vi "GUI_HTU_EMQ_triplet v2.vi"() -> ()   [LabVIEW 2020]
uses:
  Shared/GUI_Template/GUI_master/tcp_new_data_event.ctl
  Shared/GUI_Template/GUI_master/tcp new data cluster.ctl
panel:
  in  "Polarity_Switch.Ch3::1":enum16{"on", "off"}(ring) caption="Enable EMQ3"
  in  "Polarity_Switch.Ch2::1":enum16{"on", "off"}(ring) caption="Enable EMQ2"
  in  "Polarity_Switch.Ch1::1":enum16{"on", "off"}(ring) caption="Enable EMQ1"
  out "Chart":cluster{dbl, dbl, dbl}(graph)
  out "EMQ3 indicator":bool
  out "EMQ2 indicator":bool
  out "EMQ1 indicator":bool
  in  "SwitchWait":dbl=1500.0 min=0.0 max=12.0
  in  "CurrentSwitch limit":dbl=0.03 min=0.0 max=12.0
  out "Power.Ch2::1":dbl caption="Power::2" min=0.0 max=12.0
  out "Voltage.Ch2::1":dbl caption="Voltage::2" min=0.0 max=12.0
  out "Current.Ch2::1":dbl caption="Current::2" min=0.0 max=12.0
  out "Power.Ch3::1":dbl caption="Power::3" min=0.0 max=12.0
  out "Voltage.Ch3::1":dbl caption="Voltage::3" min=0.0 max=12.0
  out "Current.Ch3::1":dbl caption="Current::3" min=0.0 max=12.0
  out "Power.Ch1::1":dbl caption="Power::1" min=0.0 max=12.0
  out "Voltage.Ch1::1":dbl caption="Voltage::1" min=0.0 max=12.0
  out "Current.Ch1::1":dbl caption="Current::1" min=0.0 max=12.0
  in  "Voltage_Limit.Ch3::1":dbl caption="EMQ3 Voltage" min=0.0 max=12.0
  in  "Enable_Output.Ch3::1":enum16{"on", "off"}(ring) caption="Enable EMQ3"
  in  "Current_Limit.Ch3::1":dbl caption="EMQ3 Current" min=-10.0 max=10.0
  in  "Voltage_Limit.Ch1::1":dbl caption="EMQ1 Voltage" min=0.0 max=12.0
  in  "Voltage_Limit.Ch2::1":dbl caption="EMQ2 Voltage" min=0.0 max=12.0
  in  "Enable_Output.Ch2::1":enum16{"on", "off"}(ring) caption="Enable EMQ2"
  in  "Enable_Output.Ch1::1":enum16{"on", "off"}(ring) caption="Enable EMQ1"
  in  "Current_Limit.Ch1::1":dbl caption="EMQ1 Current" min=-10.0 max=10.0
  in  "Current_Limit.Ch2::1":dbl caption="EMQ2 Current" min=-10.0 max=10.0
  in  "UDP error message":string
  in  "GUIdevice 1":string="U_EMQTripletBipolar"
  out "error IO 2":errorcluster
  out "tcp data event":T1
  in  "stop":bool
  # "HTU EMQ Triplet"
  # "Polarity indicator"
  # "EMQ1\nEMQ1"
  # "EMQ2\nEMQ2"
  # "EMQ3"
  # "Enable output"
  # "Current Limit"
  # "Voltage Limit"
  # "Current"
  # "Voltage"
  # "Power"
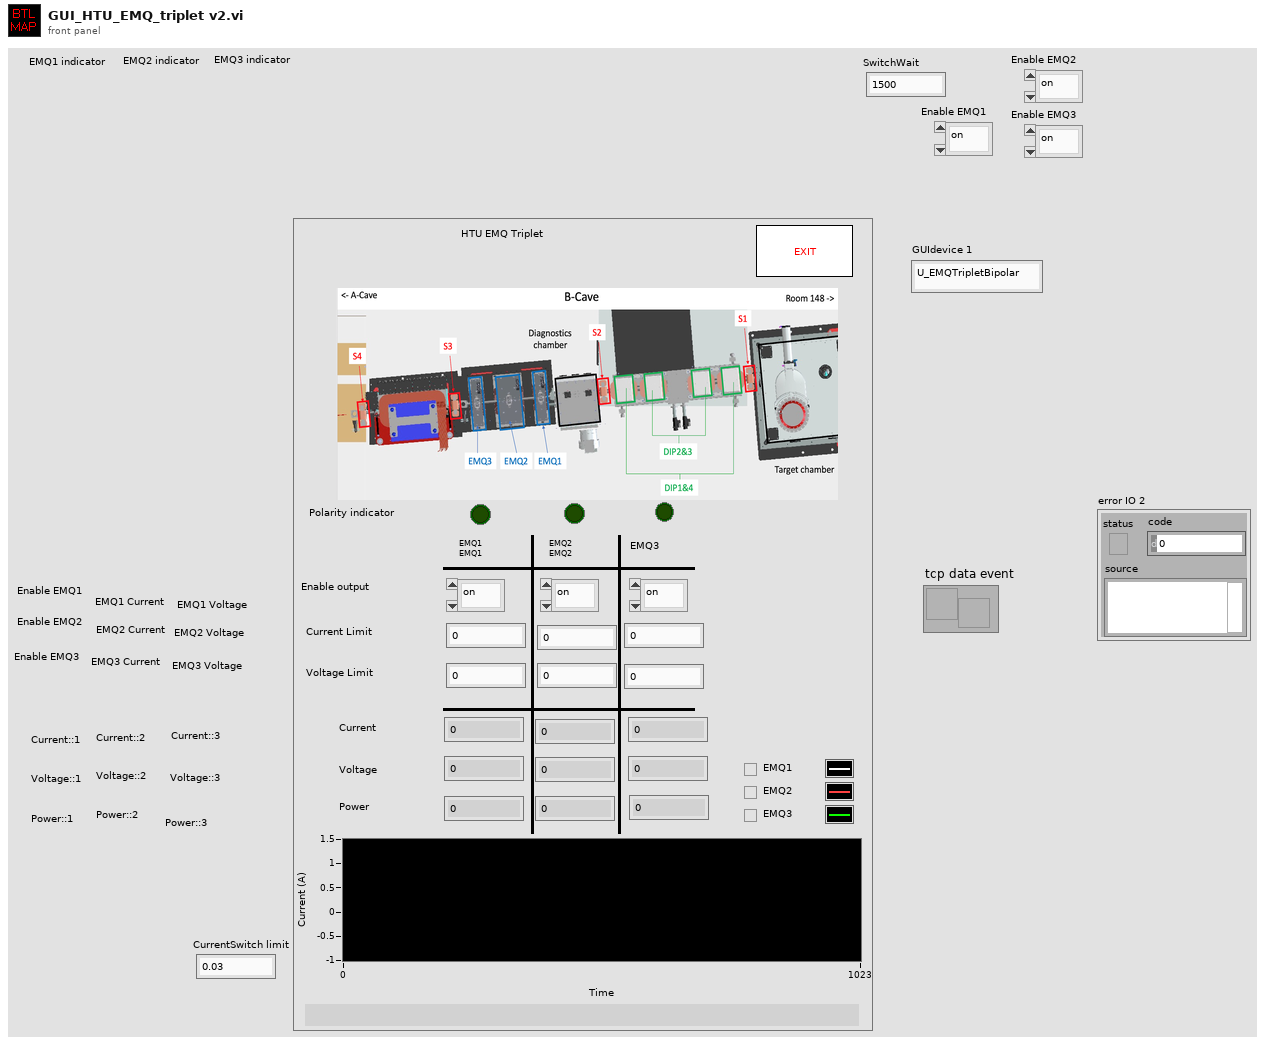
[diagram p1: front panel]
types:
  T1 = typedef "tcp_new_data_event.ctl" = refnum<user-event>
  T2 = typedef "tcp new data cluster.ctl" = cluster{"EventEnum":enum16{"new data", "connection status update"}, "Device name":string}
  T3 = enum32{"invalid app kind", "Development System", "Run Time System", "Student Edition", "Embedded LabVIEW", "Evaluation", "Custom"}
  T4 = enum32{"Invalid", "Standard", "Closed", "Hidden", "Minimized", "Maximized"}
  T5 = cluster{"Core":cluster{"Current VI Reference":refnum<vi>, "Close Panel on Exit?":bool}, "CurrentGraph1":dbl[][], "EMQ1PolaritySwitched":bool, "EMQ2PolaritySwitched":bool, "EMQ3PolaritySwitched":bool, "DegaussEMQ1":bool, "degauss loop":i32, "EMQ1DegaussSetCur":dbl, "EMQ2DegaussSetCur":dbl, "EMQ3DegaussSetCur":dbl, "last chart update tck":i32}
  T6 = cluster{"Current VI Reference":refnum<vi>, "Close Panel on Exit?":bool}
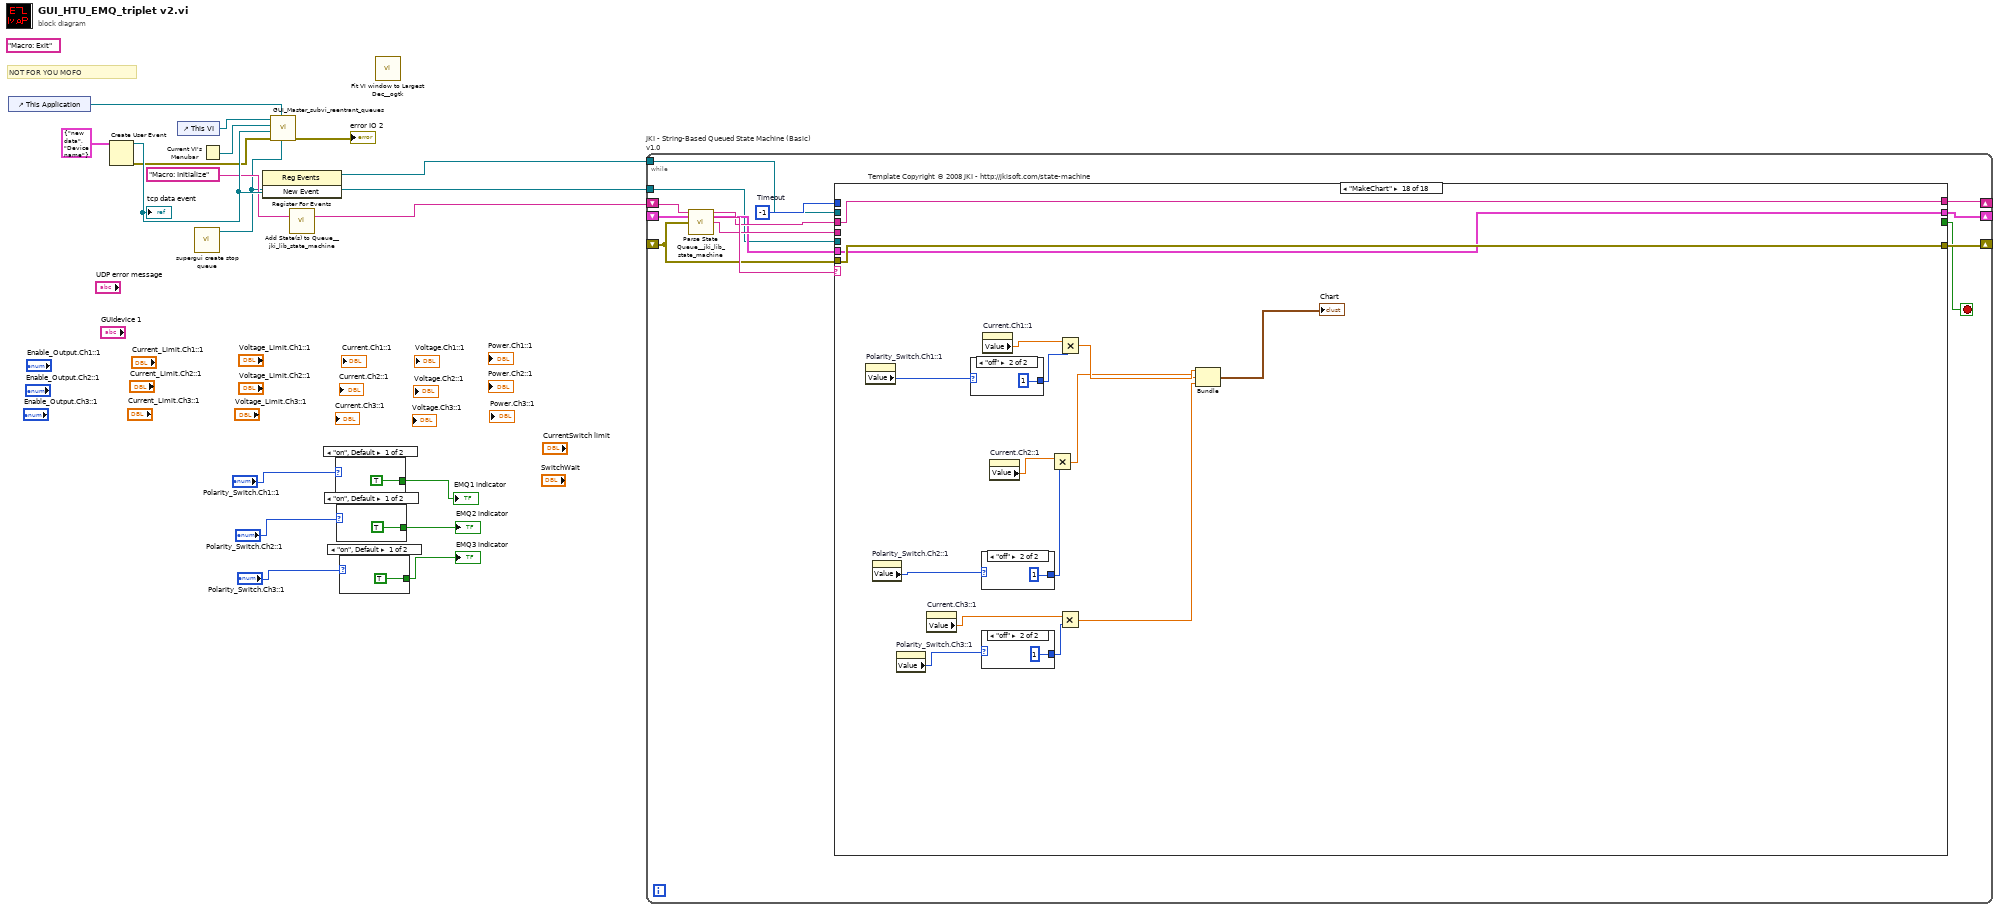
[diagram p0: block diagram]
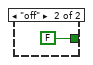
[diagram p2: hidden frame]
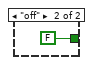
[diagram p3: hidden frame]
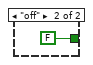
[diagram p4: hidden frame]
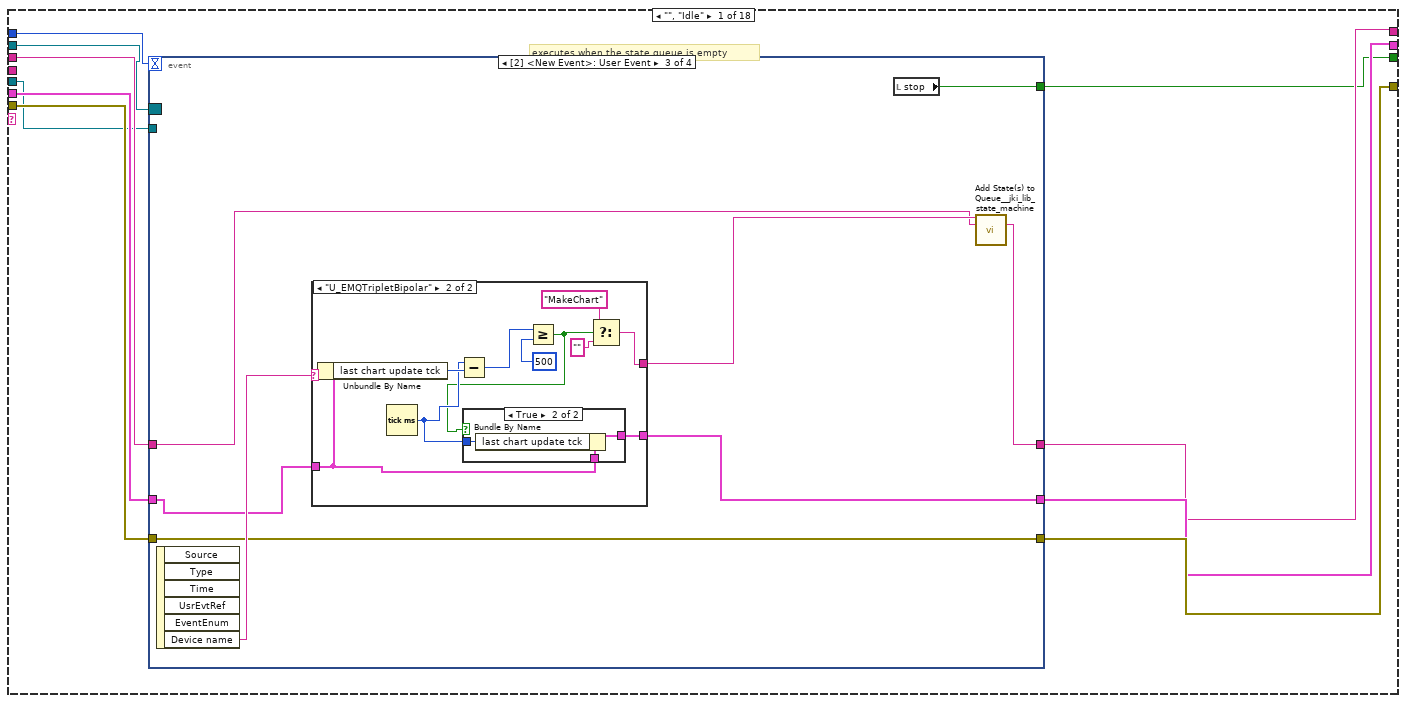
[diagram p5: hidden frame]
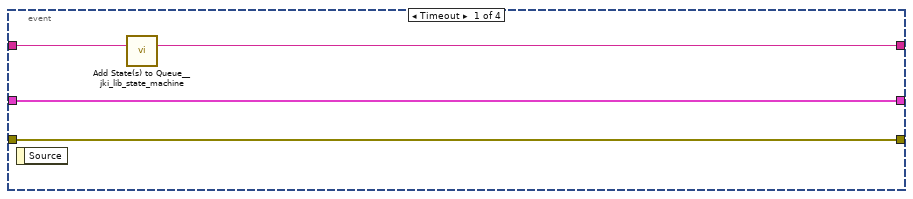
[diagram p6: hidden frame]
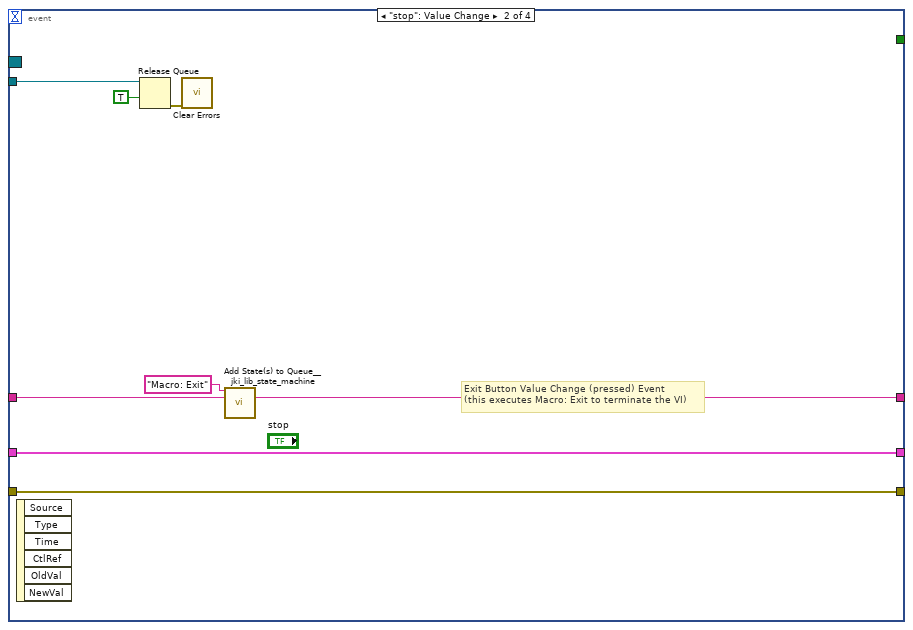
[diagram p7: hidden frame]
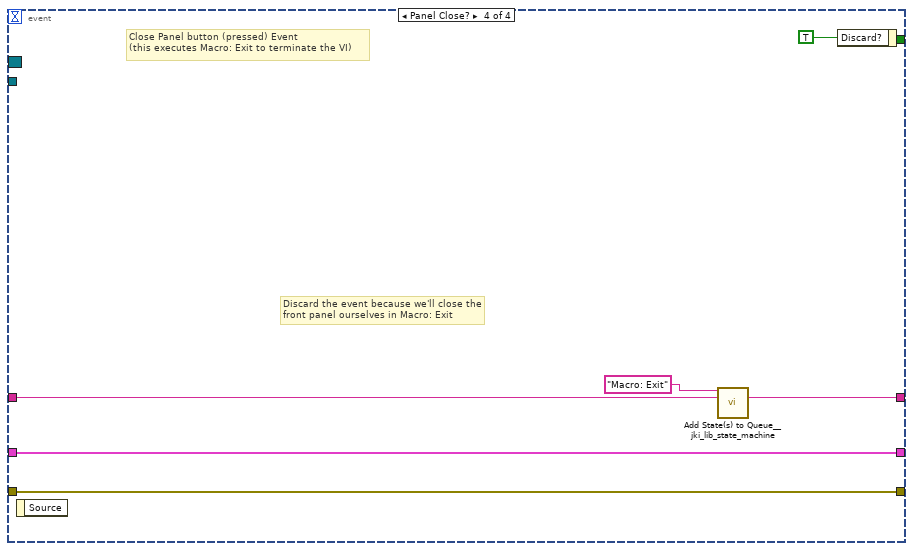
[diagram p10: hidden frame]
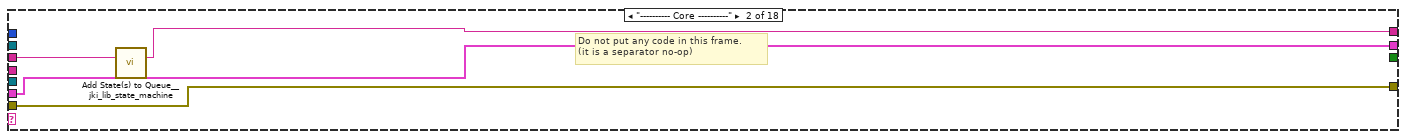
[diagram p11: hidden frame]
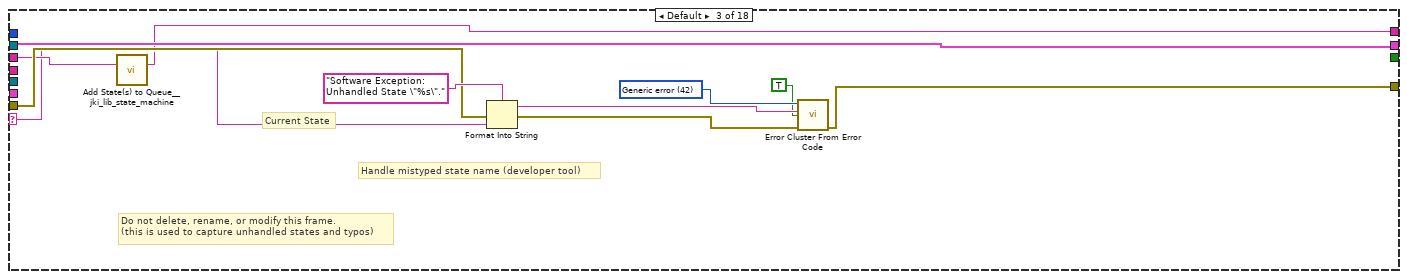
[diagram p12: hidden frame]
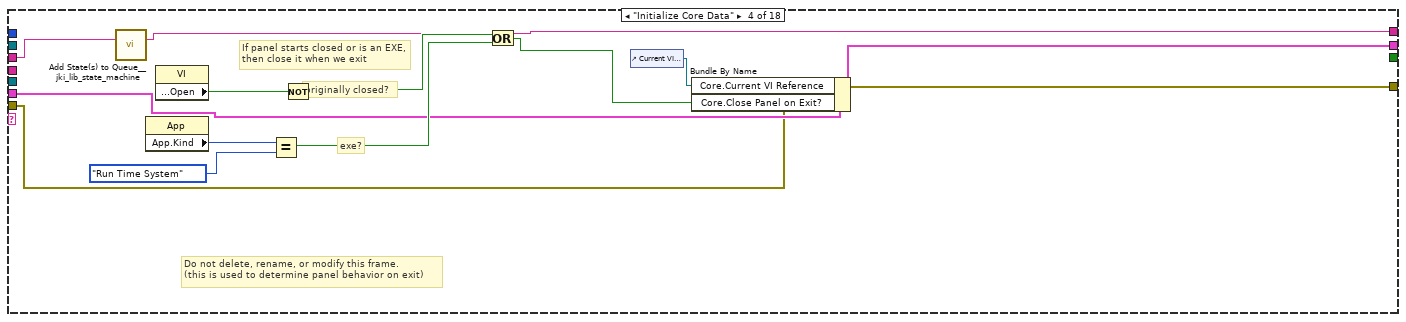
[diagram p13: hidden frame]
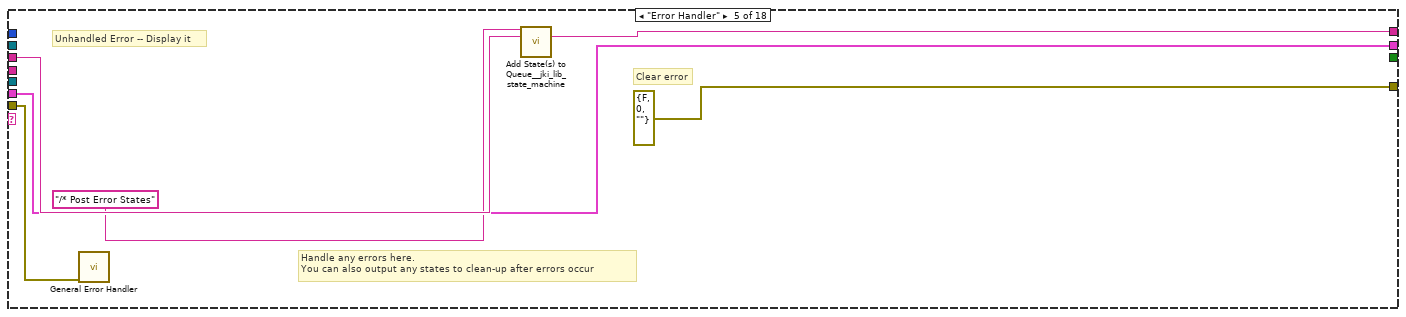
[diagram p14: hidden frame]
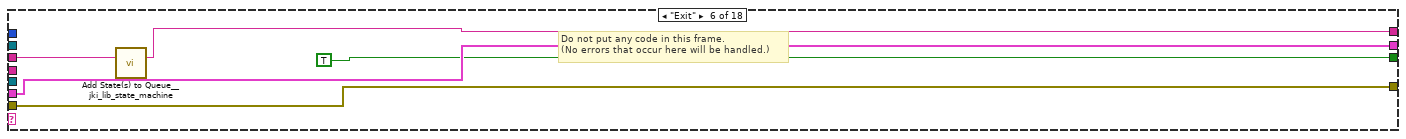
[diagram p15: hidden frame]
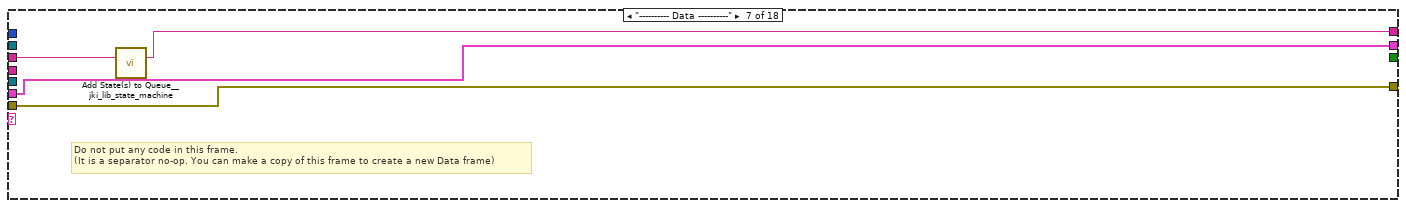
[diagram p16: hidden frame]
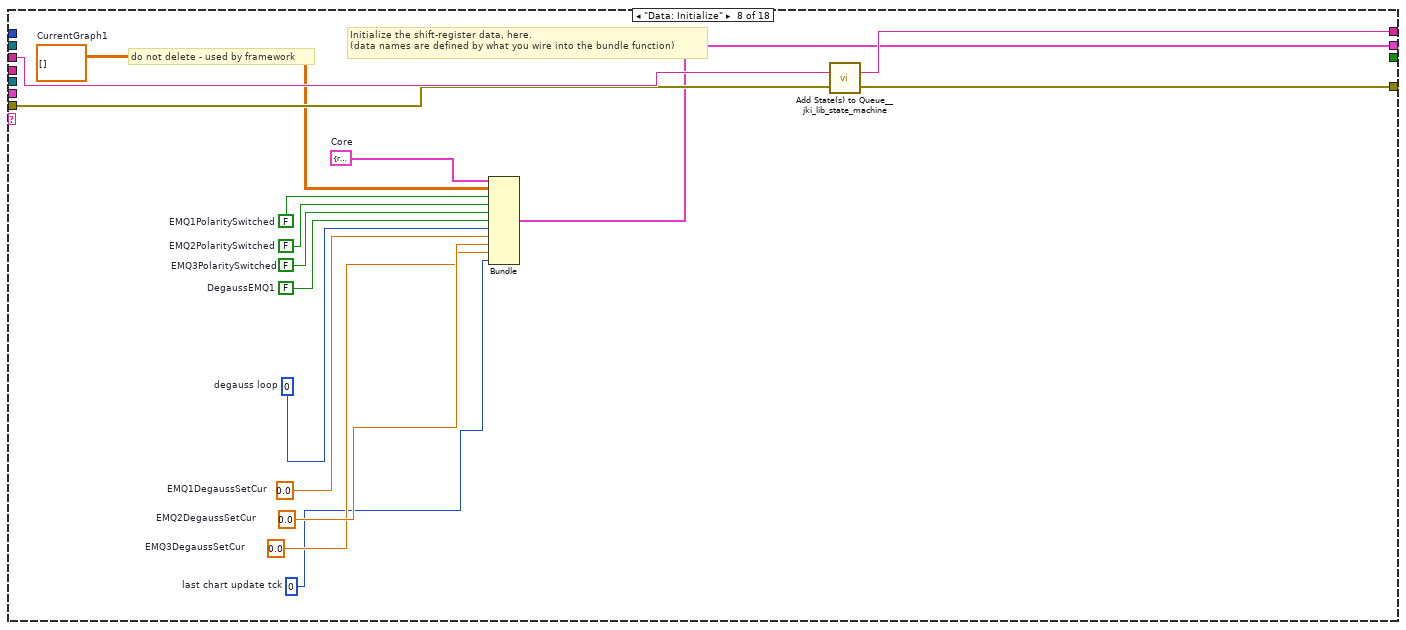
[diagram p17: hidden frame]
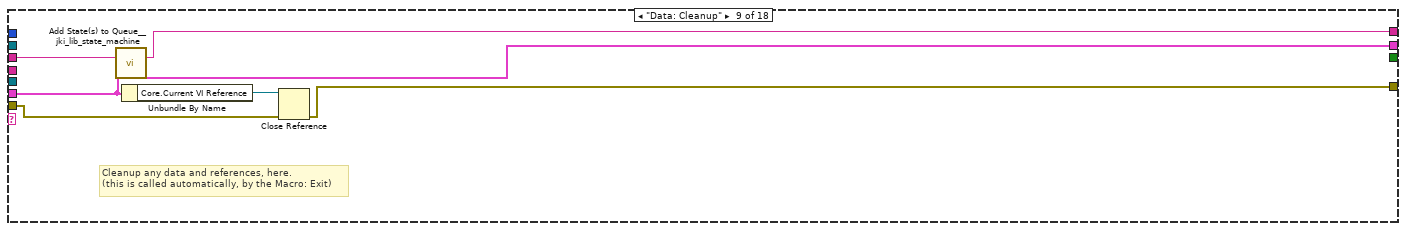
[diagram p18: hidden frame]
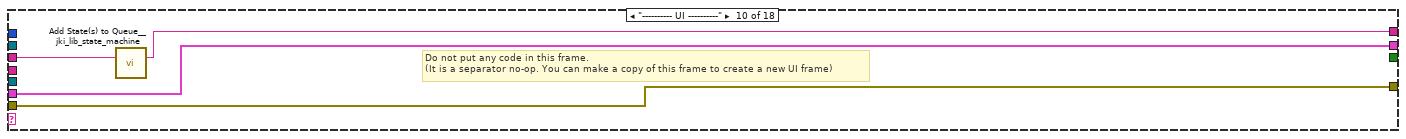
[diagram p19: hidden frame]
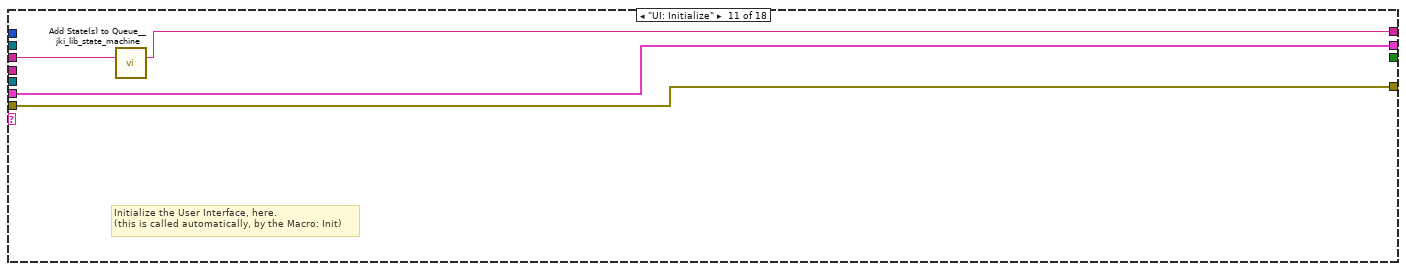
[diagram p20: hidden frame]
diagram:
  (unwired) "Macro: Exit"
  # "NOT FOR YOU MOFO"
  n1 = control-ref of="This Application"() -> (w17:refnum<vi>)
  n2 = Create User Event(user event datatype=T2 {"EventEnum"=enum."new data", "Device name"="Device name"} ("New Event")) -> (user event=w16:refnum<user-event>, error out=w15:errorcluster)  [unwired: 1 in]
  "tcp data event" <- w16
  n3 = control-ref of="This VI"() -> (w11:refnum<vi>)
  n4 = call "supergui create stop queue.vi"() -> ("STOP Queue out"=w7:refnum<queue>)  [unwired: 11 in]
  n5 = Current VI's Menubar() -> (w13:refnum<k9>)
  n6 = register-events(w16) -> (reference out=w8:refnum<event-registration>)  [unwired: 2 in, 1 out]
  n7 = call "GUI_Master_subvi_reentrant_queues.vi"("STOP Queue in"=w7, "This Application"=w17, "error in (no error)"=w15, "tcp data event"=w16, "Caller menu reference"=w13, "Caller VI ref"=w11) -> ("error out"=→"error IO 2":errorcluster)  [unwired: 5 in]
  n8 = call <vilib>:"Add State(s) to Queue__jki_lib_state_machine.vi"("State(s) in (\"\")"="Macro: Initialize") -> ("States Out"=w9:string)  [unwired: 14 in]
  n9 = case shown="\"on\", Default" "Polarity_Switch.Ch1::1" {
    tunnel: [TRUE FALSE] -> w5
    frame "on", Default {
    }
    frame "off" {
    }
  }
  "EMQ1 indicator" <- w5
  n10 = case shown="\"on\", Default" "Polarity_Switch.Ch2::1" {
    tunnel: [TRUE FALSE] -> w2
    frame "on", Default {
    }
    frame "off" {
    }
  }
  "EMQ2 indicator" <- w2
  n11 = case shown="\"on\", Default" "Polarity_Switch.Ch3::1" {
    tunnel: [TRUE FALSE] -> w1
    frame "on", Default {
    }
    frame "off" {
    }
  }
  "EMQ3 indicator" <- w1
  n12 = call <userlib>:"Fit VI window to Largest Dec__ogtk.vi"() -> ()  [unwired: 6 in, 2 out]
  n13 = while "JKI - String-Based Queued State Machine (Basic) v1.0" {
    shift-right: [w30] -> _
    shift-left: _ -> [w29]
    shift-right: [w32] -> _
    shift-left: _ -> [w27]
    shift-right: [w24] -> _
    shift-left: w9 -> [w33]
    tunnel: w8 -> [w26]
    tunnel: w7 -> [w25]
    stop <- w31 stop-if-true
    w28 = -1  # Timeout
    # "Template Copyright © 2008 JKI - http://jkisoft.com/state-machine"
    n14 = call <vilib>:"Parse State Queue__jki_lib_state_machine.vi"("State Queue"=w33, "Error In (no error)"=w27) -> ("Remaining States"=w35:string, "Current State"=w36:string, "Arguments"=w34:string)  [unwired: 11 in]
    n15 = case shown="\"MakeChart\"" w36 {
      selector: w36 -> [_ _ w93 _ _ _ _ _ _ _ _ _ _ _ _ _ _ _]
      tunnel: w35 -> [w46 w91 w96 w114 w120 w125 w129 w144 w150 w154 w158 w164 w175 w201 w206 w216 w220 w235]
      tunnel: w34 -> [_ _ _ _ _ _ _ _ _ _ _ w160 w171 _ _ _ _ _]
      tunnel: w29 -> [w45 w89 w95 w106 w119 w124 w127 _ w146 w152 w157 w163 w170 w199 w204 w208 w218 w228]
      tunnel: [w44 w90 w98 w103 errorcluster {"status"=FALSE, "code"=0, "source"=""} ("error out") w123 w128 w143 w148 w153 w156 w161 w173 w200 w205 w215 w219 w236] -> w32
      tunnel: w27 -> [w43 w90 w97 w103 w118 w123 w128 w143 w149 w153 w156 w162 w174 w200 w205 w215 w219 w236]
      tunnel: [w37 _ _ _ _ TRUE _ _ _ _ _ _ _ _ _ _ _ _] -> w31
      tunnel: [w40 w89 w95 w105 w119 w124 w127 w133 w146 w152 w157 w163 w170 w199 w204 w208 w218 w228] -> w30
      tunnel: w28 -> [w42 _ _ _ _ _ _ _ _ _ _ _ _ _ _ _ _ _]
      tunnel: w26 -> [w38 _ _ _ _ _ _ _ _ _ _ _ _ _ _ _ _ _]
      tunnel: w25 -> [w41 _ _ _ _ _ _ _ _ _ _ _ _ _ _ _ _ _]
      tunnel: [w39 w88 w92 w104 w115 w121 w126 w139 w145 w151 w155 w159 w169 w198 w202 w207 w217 w235] -> w24
      frame "", "Idle" {
        # "executes when the state queue is empty"
        n16 = event shown="[2] <New Event>: User Event" {
          selector: w38 -> [_ _ _ _]
          dyn-events: _ -> [_ _ _ _]
          timeout: w42 -> [_ _ _ _]
          tunnel: w46 -> [w50 w58 w64 w87]
          tunnel: [w49 w57 w63 w86] -> w39
          tunnel: w45 -> [w47 w55 w60 w84]
          tunnel: [w48 w56 w62 w85] -> w44
          tunnel: w43 -> [w48 w56 w62 w85]
          tunnel: [w47 w55 w59 w84] -> w40
          tunnel: w41 -> [_ w52 _ _]
          tunnel: [_ _ w61 _] -> w37
          event Timeout {
            n17 = event-data() -> ()  [unwired: 1 in, 1 out]
            n18 = call <vilib>:"Add State(s) to Queue__jki_lib_state_machine.vi"("State(s) in (\"\")"=w50) -> ("States Out"=w49:string)  [unwired: 14 in]
          }
          event "stop": Value Change {
            # "Exit Button Value Change (pressed) Event\n(this executes Macro: Exit to terminate the VI)"
            n19 = event-data() -> ()  [unwired: 1 in, 6 out]
            n20 = Release Queue(queue=w52, force destroy? (F)=TRUE) -> (error out=w53:errorcluster)  [unwired: 1 in, 2 out]
            n21 = call <vilib>:"Clear Errors.vi"("error in (no error)"=w53) -> ()  [unwired: 5 in, 2 out]
            n22 = call <vilib>:"Add State(s) to Queue__jki_lib_state_machine.vi"("State(s) in Front (\"\")"="Macro: Exit", "State(s) in (\"\")"=w58) -> ("States Out"=w57:string)  [unwired: 13 in]
          }
          event User Event {
            n23 = event-data() -> ("Device name"=w65:string)  [unwired: 1 in, 5 out]
            n24 = case shown="\"U_EMQTripletBipolar\"" w65 {
              tunnel: [_ w70] -> w66
              tunnel: w60 -> [w67 w76]
              tunnel: [w67 w77] -> w59
              frame "False", Default {
              }
              frame "U_EMQTripletBipolar" {
                n25 = Unbundle By Name(w76) -> ("last chart update tck"=w75:i32)
                n26 = Tick Count (ms)() -> (millisecond timer value=w69:u32)
                n27 = Subtract(x=w69, y=w75) -> (x-y=w74:u32)
                n28 = Greater Or Equal?(x=w74, y=u32 500 ("x")) -> (x >= y?=w68:bool)
                n29 = case shown="True" w68 {
                  tunnel: [w78 w81] -> w77
                  tunnel: w76 -> [w78 w80]
                  tunnel: w69 -> [_ w79]
                  frame False {
                  }
                  frame True {
                    n30 = Bundle By Name(cluster=w80, "last chart update tck"=w79) -> (w81:T5)
                  }
                }
                n31 = Select(t="MakeChart", s=w68, f="") -> (s? t:f=w70:string)
              }
            }
            n32 = local read "stop"() -> (w61:bool)
            n33 = call <vilib>:"Add State(s) to Queue__jki_lib_state_machine.vi"("State(s) in Front (\"\")"=w66, "State(s) in (\"\")"=w64) -> ("States Out"=w63:string)  [unwired: 13 in]
          }
          event Panel Close? {
            # "Discard the event because we'll close the front panel ourselves in Macro: Exit"
            # "Close Panel button (pressed) Event\n(this executes Macro: Exit to terminate the VI)"
            n34 = event-data() -> ()  [unwired: 1 in, 1 out]
            n35 = call <vilib>:"Add State(s) to Queue__jki_lib_state_machine.vi"("State(s) in Front (\"\")"="Macro: Exit", "State(s) in (\"\")"=w87) -> ("States Out"=w86:string)  [unwired: 13 in]
            n36 = event-data("Discard?"=TRUE) -> ()  [unwired: 1 in, 1 out]
          }
        }
      }
      frame "---------- Core ----------" {
        # "Do not put any code in this frame.\n(it is a separator no-op)"
        n37 = call <vilib>:"Add State(s) to Queue__jki_lib_state_machine.vi"("State(s) in (\"\")"=w91) -> ("States Out"=w88:string)  [unwired: 14 in]
      }
      frame Default {
        w101 = 42 items=["No error", "Argument error", "Memory is full", "Out of zone", "End of file", "File already open", "Generic file I/O error", "File not found", "File permission error", "Disk is full", "Duplicate path", "Too many files open", "System feature not enabled", "Resource file not found", "Cannot add resource", "Resource not found", "Image not found", "Image memory error", "Pen does not exist", "Config type invalid", "Config token not found", "Config parse error", "Config memory error", "Bad external code format", "Bad external code offset", "External code not present", "Null window", "Destroy window error", "Null menu", "Print aborted", "Bad print record", "Print driver error", "Windows error during printing", "Memory error during printing", "Print dialog error", "Generic print error", "Invalid device refnum", "Device not found", "Device parameter error", "Device unit error", "Cannot open device", "Device call aborted", "Generic error", "Cancelled by user", "Object ID too low", "Object ID too high", "Object not in heap", "Unknown heap", "Unknown object (invalid DefProc)", "Unknown object (DefProc not in table)", "Message out of range", "Invalid (null) method", "Unknown message", "Manager call not supported", "Bad address", "Network operation in progress", "Network operation timed out", "Connection is busy", "Network attribute not supported", "Network error", "Address in use", "System out of memory", "Connection aborted", "Connection refused", "Not connected", "Already connected", "Connection closed", "Initialization error (interapplication manager)", "Bad occurrence", "Wait on unbound occurrence handler", "Occurrence queue overflow", "Datalog type conflict", "Unused", "Unrecognized type (interapplication manager)", "Memory corrupt", "Failed to make temporary DLL", "Old CIN version", "Drag socket not found", "Failed to load drop-object", "Failed to register OLE object", "Failed to release OLE object", "Format specifier type mismatch", "Unknown format specifier", "Too few format specifiers", "Too many format specifiers", "Scan failed", "Newer CIN version", "Error converting to variant", "Runtime menu error", "Password tampered", "Variant attribute not found", "Incompatible variant data type", "Event data is not available", "Event Store is not present", "Occurrence is not found", "Event Queue is not created", "Event info is not available", "Refnum passed is NULL", "Error retrieving Class GUID", "Error retrieving CoClass GUID", "Error retrieving TypeLib GUID.", "Bad built application magic bytes.", "Specific driver is different from the specific driver associated with the Logical Name.", "There is no session opened to the class driver.", "Max Error", "MAX - Error with config objects", "MAX - Error loading configuration", "MAX - Group not supported"]
        # "Current State"
        # "Do not delete, rename, or modify this frame.\n(this is used to capture unhandled states and typos)"
        # "Handle mistyped state name (developer tool)"
        n38 = call <vilib>:"Add State(s) to Queue__jki_lib_state_machine.vi"("State(s) in (\"\")"=w96) -> ("States Out"=w92:string)  [unwired: 14 in]
        n39 = Format Into String(format string="Software Exception: Unhandled State \"%s\"." ("message"), error in=w97, w93) -> (resulting string=w100:string, error out=w99:errorcluster)  [unwired: 1 in]
        n40 = call <vilib>:"Error Cluster From Error Code.vi"("show call chain? (False)"=TRUE, "error in (no error)"=w99, "error message (\"\")"=w100, "error code (0)"=w101) -> ("error out"=w98:errorcluster)  [unwired: 5 in]
      }
      frame "Initialize Core Data" {
        # "Do not delete, rename, or modify this frame.\n(this is used to determine panel behavior on exit)"
        # "originally closed?"
        # "exe?"
        # "If panel starts closed or is an EXE, then close it when we exit"
        n41 = call <vilib>:"Add State(s) to Queue__jki_lib_state_machine.vi"("State(s) in (\"\")"=w114) -> ("States Out"=w104:string)  [unwired: 14 in]
        n42 = property class="App"() -> ("App.Kind"=w112:T3)  [unwired: 2 in, 2 out]
        n43 = property class="VI"() -> ("Front Panel.Open"=w113:bool)  [unwired: 2 in, 2 out]
        n44 = Equal?(x=w112, y=T3."Run Time System" ("Application:Kind")) -> (x = y?=w109:bool)
        n45 = Not(x=w113) -> (.not. x?=w110:bool)
        n46 = Or(x=w110, y=w109) -> (x .or. y?=w108:bool)
        n47 = control-ref of="Current VI Reference"() -> (w107:refnum<vi>)
        n48 = Bundle By Name(cluster=w106, "Core.Current VI Reference"=w107, "Core.Close Panel on Exit?"=w108) -> (w105:T5)
      }
      frame "Error Handler" {
        # "Unhandled Error -- Display it"
        # "Handle any errors here.\nYou can also output any states to clean-up after errors occur"
        # "Clear error"
        n49 = call <vilib>:"General Error Handler.vi"("error in (no error)"=w118) -> ()  [unwired: 10 in, 5 out]
        n50 = call <vilib>:"Add State(s) to Queue__jki_lib_state_machine.vi"("State(s) in Front (\"\")"="/* Post Error States", "State(s) in (\"\")"=w120) -> ("States Out"=w115:string)  [unwired: 13 in]
      }
      frame "Exit" {
        # "Do not put any code in this frame.\n(No errors that occur here will be handled.)"
        n51 = call <vilib>:"Add State(s) to Queue__jki_lib_state_machine.vi"("State(s) in (\"\")"=w125) -> ("States Out"=w121:string)  [unwired: 14 in]
      }
      frame "---------- Data ----------" {
        # "Do not put any code in this frame.\n(It is a separator no-op. You can make a copy of this frame to create a new Data frame)"
        n52 = call <vilib>:"Add State(s) to Queue__jki_lib_state_machine.vi"("State(s) in (\"\")"=w129) -> ("States Out"=w126:string)  [unwired: 14 in]
      }
      frame "Data: Initialize" {
        w130 = 0  # last chart update tck
        w131 = 0.0  # EMQ3DegaussSetCur
        w132 = 0.0  # EMQ2DegaussSetCur
        w134 = 0.0  # EMQ1DegaussSetCur
        w135 = 0  # degauss loop
        w136 = FALSE  # DegaussEMQ1
        w137 = FALSE  # EMQ3PolaritySwitched
        w138 = FALSE  # EMQ2PolaritySwitched
        w140 = FALSE  # EMQ1PolaritySwitched
        w141 = dbl[][] []  # CurrentGraph1
        w142 = T6 {"Current VI Reference"=refnum, "Close Panel on Exit?"=FALSE}  # Core
        # "do not delete - used by framework"
        # "Initialize the shift-register data, here.\n(data names are defined by what you wire into the bundle function)"
        n53 = Bundle("Core"=w142, "CurrentGraph1"=w141, "EMQ1PolaritySwitched"=w140, "EMQ2PolaritySwitched"=w138, "EMQ3PolaritySwitched"=w137, "DegaussEMQ1"=w136, "degauss loop"=w135, "EMQ1DegaussSetCur"=w134, "EMQ2DegaussSetCur"=w132, "EMQ3DegaussSetCur"=w131, "last chart update tck"=w130) -> (w133:T5)  [unwired: 1 in]
        n54 = call <vilib>:"Add State(s) to Queue__jki_lib_state_machine.vi"("State(s) in (\"\")"=w144) -> ("States Out"=w139:string)  [unwired: 14 in]
      }
      frame "Data: Cleanup" {
        # "Cleanup any data and references, here.\n(this is called automatically, by the Macro: Exit)"
        n55 = call <vilib>:"Add State(s) to Queue__jki_lib_state_machine.vi"("State(s) in (\"\")"=w150) -> ("States Out"=w145:string)  [unwired: 14 in]
        n56 = Unbundle By Name(w146) -> ("Core.Current VI Reference"=w147:refnum<vi>)
        n57 = Close Reference(reference=w147, error in (no error)=w149) -> (error out=w148:errorcluster)
      }
      frame "---------- UI ----------" {
        # "Do not put any code in this frame.\n(It is a separator no-op. You can make a copy of this frame to create a new UI frame)"
        n58 = call <vilib>:"Add State(s) to Queue__jki_lib_state_machine.vi"("State(s) in (\"\")"=w154) -> ("States Out"=w151:string)  [unwired: 14 in]
      }
      frame "UI: Initialize" {
        # "Initialize the User Interface, here.\n(this is called automatically, by the Macro: Init)"
        n59 = call <vilib>:"Add State(s) to Queue__jki_lib_state_machine.vi"("State(s) in (\"\")"=w158) -> ("States Out"=w155:string)  [unwired: 14 in]
      }
      frame "UI: Cursor Set" {
        # "Argument"
        # "Set and Unset Cursor Busy.\n(Usage: \"UI: Cursor Set >> Busy|Idle\")"
        n60 = call <vilib>:"Add State(s) to Queue__jki_lib_state_machine.vi"("State(s) in (\"\")"=w164) -> ("States Out"=w159:string)  [unwired: 14 in]
        n61 = case shown="\"Idle\", Default" w160 {
          tunnel: w162 -> [w166 w168]
          tunnel: [w165 w167] -> w161
          frame "Idle", Default {
            n62 = call <vilib>:"Unset Busy.vi"("error in (no error)"=w166) -> ("error out"=w165:errorcluster)  [unwired: 10 in]
          }
          frame "Busy" {
            n63 = call <vilib>:"Set Busy.vi"("error in (no error)"=w168) -> ("error out"=w167:errorcluster)  [unwired: 9 in, 1 out]
          }
        }
      }
      frame "UI: Front Panel State" {
        # "Argument"
        # "Set Front Panel Open or Closed\n(Usage: \"UI: Front Panel State >> Open|Close\")"
        n64 = call <vilib>:"Add State(s) to Queue__jki_lib_state_machine.vi"("State(s) in (\"\")"=w175) -> ("States Out"=w169:string)  [unwired: 14 in]
        n65 = Unbundle By Name(w170) -> ("Core.Current VI Reference"=w172:refnum<vi>)
        n66 = case shown="\"Open\", Default" w171 {
          tunnel: w174 -> [w180 w192]
          tunnel: [w181 w193] -> w173
          tunnel: w172 -> [w176 w188]
          frame "Open", Default {
            n67 = property class="VI"(reference=w176, error in=w180) -> (reference out=w178:refnum<vi>, error out=w179:errorcluster, "Front Panel.Open"=w177:bool)
            n68 = case shown="False" w177 {
              tunnel: [w184 w187] -> w181
              tunnel: w179 -> [w183 w187]
              tunnel: w178 -> [w182 _]
              frame False {
                n69 = invoke class="VI" method="FP.Open"(reference=w182, error in=w183, "Activate"=TRUE, "State"=T4."Standard") -> (error out=w184:errorcluster)  [unwired: 1 in, 4 out]
              }
              frame True {
              }
            }
          }
          frame "Close" {
            n70 = property class="VI"(reference=w188, error in=w192) -> (reference out=w190:refnum<vi>, error out=w191:errorcluster, "Front Panel.Open"=w189:bool)
            n71 = case shown="True" w189 {
              tunnel: [w194 w197] -> w193
              tunnel: w191 -> [w194 w196]
              tunnel: w190 -> [_ w195]
              frame False {
              }
              frame True {
                n72 = invoke class="VI" method="FP.Close"(reference=w195, error in=w196) -> (error out=w197:errorcluster)  [unwired: 1 in, 2 out]
              }
            }
          }
        }
      }
      frame "---------- Macro ----------" {
        # "Do not put any code in this frame.\n(It is a separator no-op. You can make a copy of this frame to create a new Macro frame)"
        n73 = call <vilib>:"Add State(s) to Queue__jki_lib_state_machine.vi"("State(s) in (\"\")"=w201) -> ("States Out"=w198:string)  [unwired: 14 in]
      }
      frame "Macro: Initialize" {
        w203 = "Data: Initialize\nInitialize Core Data\nUI: Initialize\nUI: Front Panel State >> Open"  # Data: Initialize Initialize Core Data UI: Initialize UI: Front Panel State >> Open
        # "Initialization Macro\n(This is called once, when the VI starts)"
        n74 = call <vilib>:"Add State(s) to Queue__jki_lib_state_machine.vi"("State(s) in Front (\"\")"=w203, "State(s) in (\"\")"=w206) -> ("States Out"=w202:string)  [unwired: 13 in]
      }
      frame "Macro: Exit" {
        # "Exit Macro\n(This is called once, when the VI exits)"
        n75 = Unbundle By Name(w208) -> ("Core.Close Panel on Exit?"=w209:bool)
        n76 = Select(t="UI: Front Panel State >> Close", s=w209, f="") -> (s? t:f=w212:string)
        n77 = call <vilib>:"Add State(s) to Queue__jki_lib_state_machine.vi"("State(s) in (\"\")"=w212, "State(s) at Back (\"\")"="Data: Cleanup\nExit") -> ("States Out"=w210:string)  [unwired: 13 in]
        n78 = call <vilib>:"Add State(s) to Queue__jki_lib_state_machine.vi"("State(s) in Front (\"\")"=w210, "State(s) in (\"\")"=w216) -> ("States Out"=w207:string)  [unwired: 13 in]
      }
      frame "---------- New Category ----------" {
        n79 = call <vilib>:"Add State(s) to Queue__jki_lib_state_machine.vi"("State(s) in (\"\")"=w220) -> ("States Out"=w217:string)  [unwired: 14 in]
      }
      frame "MakeChart" {
        n80 = property on="Polarity_Switch.Ch1::1" class="Enum (strict)"() -> ("Value"=w223:enum16{"on", "off"})  [unwired: 2 in, 2 out]
        n81 = property on="Polarity_Switch.Ch2::1" class="Enum (strict)"() -> ("Value"=w222:enum16{"on", "off"})  [unwired: 2 in, 2 out]
        n82 = property on="Polarity_Switch.Ch3::1" class="Enum (strict)"() -> ("Value"=w221:enum16{"on", "off"})  [unwired: 2 in, 2 out]
        n83 = property on="Current.Ch3::1" class="DigNum (strict)"() -> ("Value"=w230:dbl)  [unwired: 2 in, 2 out]
        n84 = case shown="\"off\"" w223 {
          tunnel: [-1 1] -> w231
          frame "on", Default {
          }
          frame "off" {
          }
        }
        n85 = case shown="\"off\"" w222 {
          tunnel: [-1 1] -> w234
          frame "on", Default {
          }
          frame "off" {
          }
        }
        n86 = case shown="\"off\"" w221 {
          tunnel: [-1 1] -> w229
          frame "on", Default {
          }
          frame "off" {
          }
        }
        n87 = property on="Current.Ch1::1" class="DigNum (strict)"() -> ("Value"=w232:dbl)  [unwired: 2 in, 2 out]
        n88 = property on="Current.Ch2::1" class="DigNum (strict)"() -> ("Value"=w233:dbl)  [unwired: 2 in, 2 out]
        n89 = Multiply(x=w233, y=w234) -> (x*y=w226:dbl)
        n90 = Multiply(x=w230, y=w229) -> (x*y=w225:dbl)
        n91 = Multiply(x=w232, y=w231) -> (x*y=w227:dbl)
        n92 = Bundle(w227, w226, w225) -> (→"Chart":cluster{dbl, dbl, dbl})  [unwired: 1 in]
      }
    }
  }
